vi "invisible cursors pos..vi"(8 "error in (no error)":errorcluster, 11 "XYGraph in":refnum<vi>) -> (0 "error out":errorcluster)   [LabVIEW 2014]
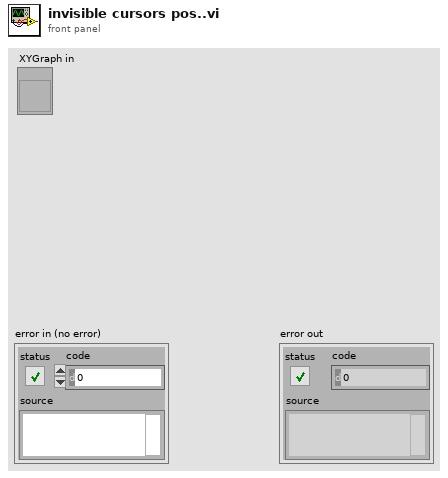
[diagram p1: front panel]
types:
  T1 = enum16{"read", "write", "write number of cursors per plot only"}
  T2 = cluster{"plot 1 cursors visible? ":bool, "plot 2 cursors visible?":bool, "plot 3 cursors visible?":bool, "No of cursors per plot":i32}
  T3 = typedef "LVCursorListTypeDef.ctl" = cluster{"Name":string, "Color":u32, "Style":u8, "Point Style":u8, "Name Visible":bool, "Allow Drag":bool, "Cursor Mode":u32, "Plot":i32, "Index":i32, "Position":cluster{"X":dbl, "Y":dbl}, "X Scale":u32, "Y Scale":u32, "Watch Plots":i32[], "Watch All Plots":bool, "Plot Area":i32, "Label Offset":cluster{"X":dbl, "Y":dbl}}[]
  T4 = cluster{"Name":string, "Color":u32, "Style":u8, "Point Style":u8, "Name Visible":bool, "Allow Drag":bool, "Cursor Mode":u32, "Plot":i32, "Index":i32, "Position":cluster{"X":dbl, "Y":dbl}, "X Scale":u32, "Y Scale":u32, "Watch Plots":i32[], "Watch All Plots":bool, "Plot Area":i32, "Label Offset":cluster{"X":dbl, "Y":dbl}}
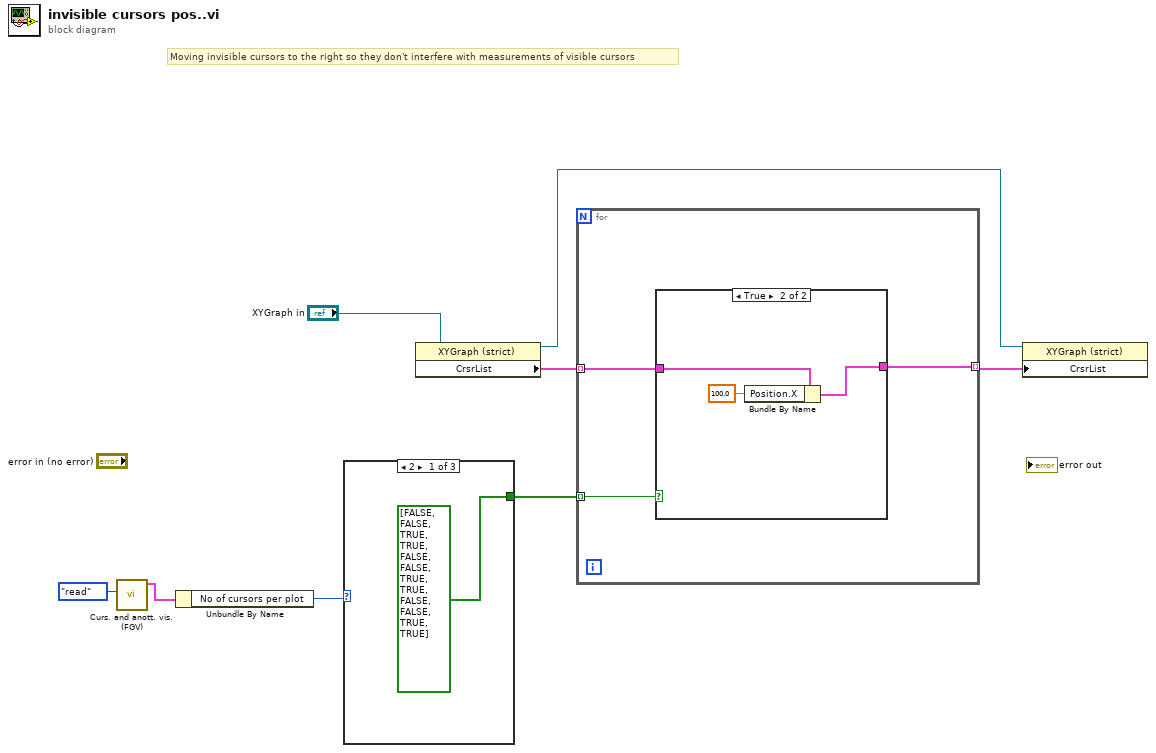
[diagram p0: block diagram]
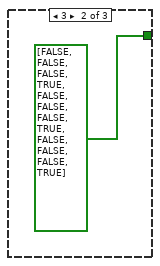
[diagram p2: hidden frame]
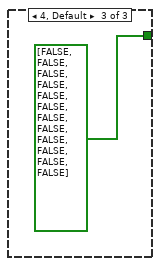
[diagram p3: hidden frame]
diagram:
  # "Moving invisible cursors to the right so they don't interfere with measurements of visible cursors"
  n1 = call "Curs. and anott. vis. (FGV).vi"("Enum"=T1."read") -> ("cursors visibility out"=w5:T2)  [unwired: 8 in, 2 out]
  n2 = Unbundle By Name(w5) -> ("No of cursors per plot"=w4:i32)
  n3 = case shown="2" w4 {
    tunnel: [bool[] [FALSE, FALSE, TRUE, TRUE, FALSE, FALSE, TRUE, TRUE, FALSE, FALSE, TRUE, TRUE] bool[] [FALSE, FALSE, FALSE, TRUE, FALSE, FALSE, FALSE, TRUE, FALSE, FALSE, FALSE, TRUE] bool[] [FALSE, FALSE, FALSE, FALSE, FALSE, FALSE, FALSE, FALSE, FALSE, FALSE, FALSE, FALSE]] -> w3
    frame 2 {
    }
    frame 3 {
    }
    frame 4, Default {
    }
  }
  n4 = property class="XYGraph (strict)"(reference="XYGraph in") -> (reference out=w2:refnum<vi>, "CrsrList"=w7:T3)  [unwired: 1 in, 1 out]
  n5 = for {
    tunnel: w7 -> [w13] mode=indexing
    tunnel: w3 -> [w14] mode=indexing
    tunnel: [w12] -> w1 mode=indexing
    n6 = case shown="True" w14 {
      tunnel: w13 -> [w15 w18]
      tunnel: [w15 w16] -> w12
      frame False {
      }
      frame True {
        n7 = Bundle By Name(cluster=w18, "Position.X"=100.0) -> (w16:T4)
      }
    }
  }
  n8 = property class="XYGraph (strict)"(reference=w2, "CrsrList"=w1) -> ()  [unwired: 1 in, 2 out]
